vi "VciEnumDeviceNext.vi"(3 "error in":errorcluster {"code" format="%.0x"}, 5 "Enum Handle in":u32 format="%x") -> (0 "error out":errorcluster {"code" format="%.0x"}, 1 "Device Info":T1 {"Unique Hardware ID"."D48" format="%02x"; "Unique Hardware ID"."D47" format="%02x"; "Unique Hardware ID"."D46" format="%02x"; "Unique Hardware ID"."D45" format="%02x"; "Unique Hardware ID"."D44" format="%02x"; "Unique Hardware ID"."D43" format="%02x"; "Unique Hardware ID"."D42" format="%02x"; "Unique Hardware ID"."D41" format="%02x"; "Unique Hardware ID"."D3" format="%04x"; "Unique Hardware ID"."D2" format="%04x"; "Unique Hardware ID"."D1" format="%08x"; "Unique VCI Object ID"."High Part" format="%08x"; "Unique VCI Object ID"."Low Part" format="%08x"; "Device Class ID"."D48" format="%02x"; "Device Class ID"."D47" format="%02x"; "Device Class ID"."D46" format="%02x"; "Device Class ID"."D45" format="%02x"; "Device Class ID"."D44" format="%02x"; "Device Class ID"."D43" format="%02x"; "Device Class ID"."D42" format="%02x"; "Device Class ID"."D41" format="%02x"; "Device Class ID"."D3" format="%04x"; "Device Class ID"."D2" format="%04x"; "Device Class ID"."D1" format="%08x"}, 2 "Enum Handle out":u32 format="%x")   [LabVIEW 2011]
doc: "Retrieves the next available VCI device."
uses:
  vcilva.dll
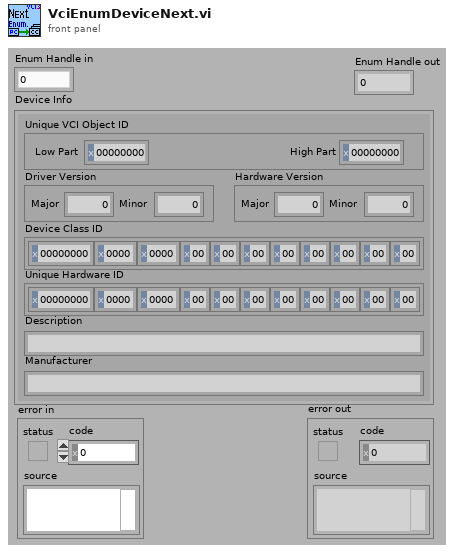
[diagram p1: front panel]
types:
  T1 = cluster{"Unique VCI Object ID":cluster{"Low Part":u32, "High Part":u32}, "Driver Version":cluster{"Major":u16, "Minor":u16}, "Hardware Version":cluster{"Major":u16, "Minor":u16}, "Device Class ID":cluster{"D1":u32, "D2":u16, "D3":u16, "D41":u8, "D42":u8, "D43":u8, "D44":u8, "D45":u8, "D46":u8, "D47":u8, "D48":u8}, "Unique Hardware ID":cluster{"D1":u32, "D2":u16, "D3":u16, "D41":u8, "D42":u8, "D43":u8, "D44":u8, "D45":u8, "D46":u8, "D47":u8, "D48":u8}, "Description":string, "Manufacturer":string}
  T2 = cluster{"Unique VCI Object ID":cluster{"Low Part":u32, "High Part":u32}, "Driver Version":cluster{"Major":u16, "Minor":u16}, "Hardware Version":cluster{"Major":u16, "Minor":u16}, "Device Class ID":cluster{"D1":u32, "D2":u16, "D3":u16, "D41":u8, "D42":u8, "D43":u8, "D44":u8, "D45":u8, "D46":u8, "D47":u8, "D48":u8}, "Unique Hardware ID":cluster{"D1":u32, "D2":u16, "D3":u16, "D41":u8, "D42":u8, "D43":u8, "D44":u8, "D45":u8, "D46":u8, "D47":u8, "D48":u8}}
  T3 = cluster{"D1":u32, "D2":u16, "D3":u16, "D41":u8, "D42":u8, "D43":u8, "D44":u8, "D45":u8, "D46":u8, "D47":u8, "D48":u8}
  T4 = cluster{"Unique VCI Object ID":cluster{"Low Part":u32, "High Part":u32}, "Driver Version":cluster{"Major":u16, "Minor":u16}, "Hardware Version":cluster{"Major":u16, "Minor":u16}, "Device Class ID":cluster{"D1":u32, "D2":u16, "D3":u16, "D41":u8, "D42":u8, "D43":u8, "D44":u8, "D45":u8, "D46":u8, "D47":u8, "D48":u8}, "Unique Hardware ID":cluster{"D1":u32, "D2":u16, "D3":u16, "D41":u8, "D42":u8, "D43":u8, "D44":u8, "D45":u8, "D46":u8, "D47":u8, "D48":u8}, string, string}
  T5 = cluster{"[0]":u8, "[1]":u8, "[2]":u8, "[3]":u8, "[4]":u8, "[5]":u8, "[6]":u8, "[7]":u8, "[8]":u8, "[9]":u8, "[10]":u8, "[11]":u8, "[12]":u8, "[13]":u8, "[14]":u8, "[15]":u8, "[16]":u8, "[17]":u8, "[18]":u8, "[19]":u8, "[20]":u8, "[21]":u8, "[22]":u8, "[23]":u8, "[24]":u8, "[25]":u8, "[26]":u8, "[27]":u8, "[28]":u8, "[29]":u8, "[30]":u8, "[31]":u8, "[32]":u8, "[33]":u8, "[34]":u8, "[35]":u8, "[36]":u8, "[37]":u8, "[38]":u8, "[39]":u8, "[40]":u8, "[41]":u8, "[42]":u8, "[43]":u8, "[44]":u8, "[45]":u8, "[46]":u8, "[47]":u8, "[48]":u8, "[49]":u8, "[50]":u8, "[51]":u8, "[52]":u8, "[53]":u8, "[54]":u8, "[55]":u8, "[56]":u8, "[57]":u8, "[58]":u8, "[59]":u8, "[60]":u8, "[61]":u8, "[62]":u8, "[63]":u8, "[64]":u8, "[65]":u8, "[66]":u8, "[67]":u8, "[68]":u8, "[69]":u8, "[70]":u8, "[71]":u8, "[72]":u8, "[73]":u8, "[74]":u8, "[75]":u8, "[76]":u8, "[77]":u8, "[78]":u8, "[79]":u8, "[80]":u8, "[81]":u8, "[82]":u8, "[83]":u8, "[84]":u8, "[85]":u8, "[86]":u8, "[87]":u8, "[88]":u8, "[89]":u8, "[90]":u8, "[91]":u8, "[92]":u8, "[93]":u8, "[94]":u8, "[95]":u8, "[96]":u8, "[97]":u8, "[98]":u8, "[99]":u8, "[100]":u8, "[101]":u8, "[102]":u8, "[103]":u8, "[104]":u8, "[105]":u8, "[106]":u8, "[107]":u8, "[108]":u8, "[109]":u8, "[110]":u8, "[111]":u8, "[112]":u8, "[113]":u8, "[114]":u8, "[115]":u8, "[116]":u8, "[117]":u8, "[118]":u8, "[119]":u8, "[120]":u8, "[121]":u8, "[122]":u8, "[123]":u8, "[124]":u8, "[125]":u8, "[126]":u8, "[127]":u8}
  T6 = cluster{"Unique VCI Object ID":cluster{"Low Part":u32, "High Part":u32}, "Driver Version":cluster{"Major":u16, "Minor":u16}, "Hardware Version":cluster{"Major":u16, "Minor":u16}, "Device Class ID":cluster{"D1":u32, "D2":u16, "D3":u16, "D41":u8, "D42":u8, "D43":u8, "D44":u8, "D45":u8, "D46":u8, "D47":u8, "D48":u8}, "Unique Hardware ID":cluster{"D1":u32, "D2":u16, "D3":u16, "D41":u8, "D42":u8, "D43":u8, "D44":u8, "D45":u8, "D46":u8, "D47":u8, "D48":u8}, cluster{"[0]":u8, "[1]":u8, "[2]":u8, "[3]":u8, "[4]":u8, "[5]":u8, "[6]":u8, "[7]":u8, "[8]":u8, "[9]":u8, "[10]":u8, "[11]":u8, "[12]":u8, "[13]":u8, "[14]":u8, "[15]":u8, "[16]":u8, "[17]":u8, "[18]":u8, "[19]":u8, "[20]":u8, "[21]":u8, "[22]":u8, "[23]":u8, "[24]":u8, "[25]":u8, "[26]":u8, "[27]":u8, "[28]":u8, "[29]":u8, "[30]":u8, "[31]":u8, "[32]":u8, "[33]":u8, "[34]":u8, "[35]":u8, "[36]":u8, "[37]":u8, "[38]":u8, "[39]":u8, "[40]":u8, "[41]":u8, "[42]":u8, "[43]":u8, "[44]":u8, "[45]":u8, "[46]":u8, "[47]":u8, "[48]":u8, "[49]":u8, "[50]":u8, "[51]":u8, "[52]":u8, "[53]":u8, "[54]":u8, "[55]":u8, "[56]":u8, "[57]":u8, "[58]":u8, "[59]":u8, "[60]":u8, "[61]":u8, "[62]":u8, "[63]":u8, "[64]":u8, "[65]":u8, "[66]":u8, "[67]":u8, "[68]":u8, "[69]":u8, "[70]":u8, "[71]":u8, "[72]":u8, "[73]":u8, "[74]":u8, "[75]":u8, "[76]":u8, "[77]":u8, "[78]":u8, "[79]":u8, "[80]":u8, "[81]":u8, "[82]":u8, "[83]":u8, "[84]":u8, "[85]":u8, "[86]":u8, "[87]":u8, "[88]":u8, "[89]":u8, "[90]":u8, "[91]":u8, "[92]":u8, "[93]":u8, "[94]":u8, "[95]":u8, "[96]":u8, "[97]":u8, "[98]":u8, "[99]":u8, "[100]":u8, "[101]":u8, "[102]":u8, "[103]":u8, "[104]":u8, "[105]":u8, "[106]":u8, "[107]":u8, "[108]":u8, "[109]":u8, "[110]":u8, "[111]":u8, "[112]":u8, "[113]":u8, "[114]":u8, "[115]":u8, "[116]":u8, "[117]":u8, "[118]":u8, "[119]":u8, "[120]":u8, "[121]":u8, "[122]":u8, "[123]":u8, "[124]":u8, "[125]":u8, "[126]":u8, "[127]":u8}, cluster{"[0]":u8, "[1]":u8, "[2]":u8, "[3]":u8, "[4]":u8, "[5]":u8, "[6]":u8, "[7]":u8, "[8]":u8, "[9]":u8, "[10]":u8, "[11]":u8, "[12]":u8, "[13]":u8, "[14]":u8, "[15]":u8, "[16]":u8, "[17]":u8, "[18]":u8, "[19]":u8, "[20]":u8, "[21]":u8, "[22]":u8, "[23]":u8, "[24]":u8, "[25]":u8, "[26]":u8, "[27]":u8, "[28]":u8, "[29]":u8, "[30]":u8, "[31]":u8, "[32]":u8, "[33]":u8, "[34]":u8, "[35]":u8, "[36]":u8, "[37]":u8, "[38]":u8, "[39]":u8, "[40]":u8, "[41]":u8, "[42]":u8, "[43]":u8, "[44]":u8, "[45]":u8, "[46]":u8, "[47]":u8, "[48]":u8, "[49]":u8, "[50]":u8, "[51]":u8, "[52]":u8, "[53]":u8, "[54]":u8, "[55]":u8, "[56]":u8, "[57]":u8, "[58]":u8, "[59]":u8, "[60]":u8, "[61]":u8, "[62]":u8, "[63]":u8, "[64]":u8, "[65]":u8, "[66]":u8, "[67]":u8, "[68]":u8, "[69]":u8, "[70]":u8, "[71]":u8, "[72]":u8, "[73]":u8, "[74]":u8, "[75]":u8, "[76]":u8, "[77]":u8, "[78]":u8, "[79]":u8, "[80]":u8, "[81]":u8, "[82]":u8, "[83]":u8, "[84]":u8, "[85]":u8, "[86]":u8, "[87]":u8, "[88]":u8, "[89]":u8, "[90]":u8, "[91]":u8, "[92]":u8, "[93]":u8, "[94]":u8, "[95]":u8, "[96]":u8, "[97]":u8, "[98]":u8, "[99]":u8, "[100]":u8, "[101]":u8, "[102]":u8, "[103]":u8, "[104]":u8, "[105]":u8, "[106]":u8, "[107]":u8, "[108]":u8, "[109]":u8, "[110]":u8, "[111]":u8, "[112]":u8, "[113]":u8, "[114]":u8, "[115]":u8, "[116]":u8, "[117]":u8, "[118]":u8, "[119]":u8, "[120]":u8, "[121]":u8, "[122]":u8, "[123]":u8, "[124]":u8, "[125]":u8, "[126]":u8, "[127]":u8}}
  T7 = cluster{"Unique VCI Object ID":cluster{"Low Part":u32, "High Part":u32}, "Driver Version":cluster{"Major":u16, "Minor":u16}, "Hardware Version":cluster{"Major":u16, "Minor":u16}, "Device Class ID":cluster{"D1":u32, "D2":u16, "D3":u16, "D41":u8, "D42":u8, "D43":u8, "D44":u8, "D45":u8, "D46":u8, "D47":u8, "D48":u8}, "Unique Hardware ID":cluster{"D1":u32, "D2":u16, "D3":u16, "D41":u8, "D42":u8, "D43":u8, "D44":u8, "D45":u8, "D46":u8, "D47":u8, "D48":u8}, "string":string, "string":string}
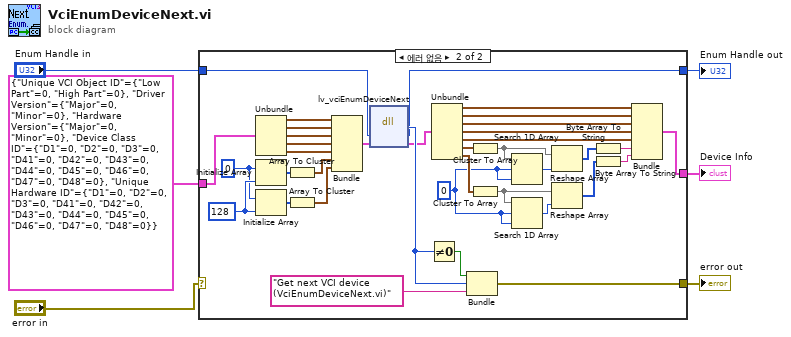
[diagram p0: block diagram]
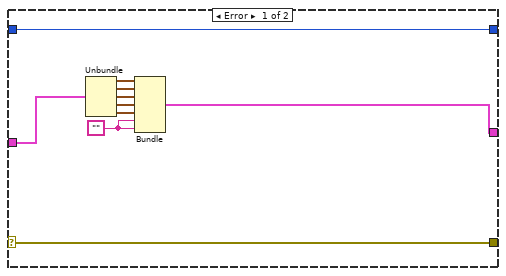
[diagram p2: hidden frame]
diagram:
  n1 = case shown="에러 없음" "error in" {
    selector: "error in" -> [w16 _]
    tunnel: [w16 w53] -> w5
    tunnel: "Enum Handle in" -> [w15 w17]
    tunnel: T2 {"Unique VCI Object ID"={"Low Part"=0, "High Part"=0}, "Driver Version"={"Major"=0, "Minor"=0}, "Hardware Version"={"Major"=0, "Minor"=0}, "Device Class ID"={"D1"=0, "D2"=0, "D3"=0, "D41"=0, "D42"=0, "D43"=0, "D44"=0, "D45"=0, "D46"=0, "D47"=0, "D48"=0}, "Unique Hardware ID"={"D1"=0, "D2"=0, "D3"=0, "D41"=0, "D42"=0, "D43"=0, "D44"=0, "D45"=0, "D46"=0, "D47"=0, "D48"=0}} ("DeviceInfo") -> [w14 w36]
    tunnel: [w15 w49] -> w4
    tunnel: [w7 w18] -> w3
    frame Error {
      w8 = ""
      n2 = Unbundle(w14) -> ("Unique VCI Object ID"=w13:cluster{"Low Part":u32, "High Part":u32}, "Driver Version"=w12:cluster{"Major":u16, "Minor":u16}, "Hardware Version"=w11:cluster{"Major":u16, "Minor":u16}, "Device Class ID"=w10:T3, "Unique Hardware ID"=w9:T3)
      n3 = Bundle("Unique VCI Object ID"=w13, "Driver Version"=w12, "Hardware Version"=w11, "Device Class ID"=w10, "Unique Hardware ID"=w9, w8, w8) -> (w7:T4)  [unwired: 1 in]
    }
    frame No Error {
      w20 = u8 0 ("element")
      w44 = u8 0 ("element")
      w45 = 128 ("dimension size")
      n4 = Unbundle(w36) -> ("Unique VCI Object ID"=w38:cluster{"Low Part":u32, "High Part":u32}, "Driver Version"=w39:cluster{"Major":u16, "Minor":u16}, "Hardware Version"=w40:cluster{"Major":u16, "Minor":u16}, "Device Class ID"=w41:T3, "Unique Hardware ID"=w42:T3)
      n5 = Initialize Array(w44, w45) -> (w43:u8[])
      n6 = Initialize Array(w44, w45) -> (w46:u8[])
      n7 = Array To Cluster(array=w43) -> (cluster=w47:T5)
      n8 = Array To Cluster(array=w46) -> (cluster=w48:T5)
      n9 = Bundle("Unique VCI Object ID"=w38, "Driver Version"=w39, "Hardware Version"=w40, "Device Class ID"=w41, "Unique Hardware ID"=w42, w47, w48) -> (w37:T6)  [unwired: 1 in]
      n10 = dll-call lib="vcilva.dll" fn="lv_vciEnumDeviceNext"("hEnum"=w17, w37) -> (w50:i32, "hEnum"=w49:u32, w21:T6)  [unwired: 3 in, 2 out]
      n11 = Not Equal To 0?(x=w50) -> (x != 0?=w52:bool)
      n12 = Unbundle(w21) -> ("Unique VCI Object ID"=w23:cluster{"Low Part":u32, "High Part":u32}, "Driver Version"=w24:cluster{"Major":u16, "Minor":u16}, "Hardware Version"=w25:cluster{"Major":u16, "Minor":u16}, "Device Class ID"=w26:T3, "Unique Hardware ID"=w27:T3, w22:T5, w28:T5)
      n13 = Bundle(w52, w50, "Get next VCI device (VciEnumDeviceNext.vi)") -> (w53:errorcluster)  [unwired: 1 in]
      n14 = Cluster To Array(cluster=w22) -> (array=w31:u8[])
      n15 = Cluster To Array(cluster=w28) -> (array=w34:u8[])
      n16 = Search 1D Array(1D array=w31, element=w20, start index (0)=w20) -> (index of element=w30:i32)
      n17 = Search 1D Array(1D array=w34, element=w20, start index (0)=w20) -> (index of element=w19:i32)
      n18 = Reshape Array(w31, w30) -> (w32:u8[])
      n19 = Reshape Array(w34, w19) -> (w35:u8[])
      n20 = Byte Array To String(unsigned byte array=w32) -> (string=w33:string)
      n21 = Byte Array To String(unsigned byte array=w35) -> (string=w29:string)
      n22 = Bundle("Unique VCI Object ID"=w23, "Driver Version"=w24, "Hardware Version"=w25, "Device Class ID"=w26, "Unique Hardware ID"=w27, "string"=w33, "string"=w29) -> (w18:T7)  [unwired: 1 in]
    }
  }
  "error out" <- w5
  "Enum Handle out" <- w4
  "Device Info" <- w3
